vi "ClipCursor to PlotArea.vi"(7 "OriginPane":refnum<vi>, 8 "error in (no error)":errorcluster, 9 "VI":refnum<vi>, 10 "PlotPane":refnum<vi>, 11 "plot ref":refnum<vi>) -> (0 "error out":errorcluster)   [LabVIEW 2021, in "RocketPlot.lvlib"]
uses:
  RocketPlot.lvlib
  <vilib>/Utility/miscctls.llb/LVPointTypeDef.ctl
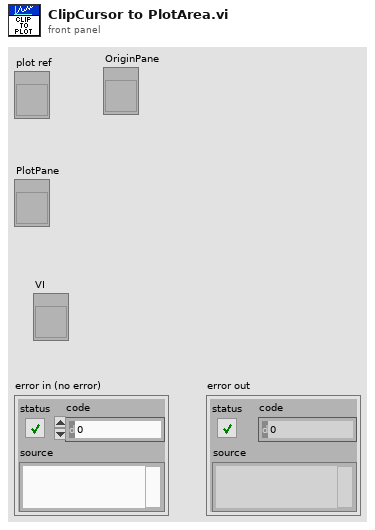
[diagram p1: front panel]
types:
  T1 = typedef "LVPointTypeDef.ctl" = cluster{"Horizontal":i16, "Vertical":i16}
  T2 = cluster{"Left":i32, "Top":i32, "Right":i32, "Bottom":i32}
  T3 = typedef "LVRectTypeDef.ctl" = cluster{"Left":i16, "Top":i16, "Right":i16, "Bottom":i16}
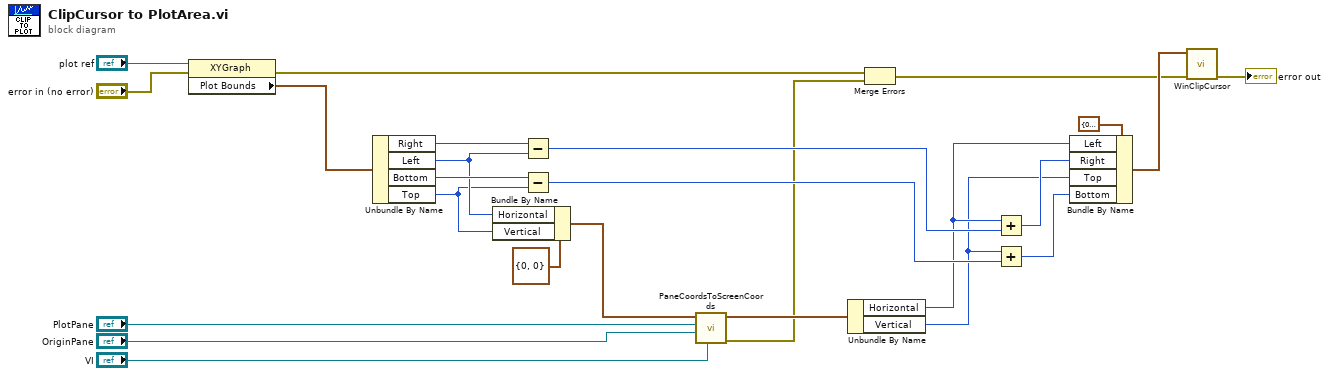
[diagram p0: block diagram]
diagram:
  n1 = property class="XYGraph"(reference="plot ref", error in="error in (no error)") -> (error out=w8:errorcluster, "Plot Bounds"=w24:T3)  [unwired: 1 out]
  n2 = Unbundle By Name(w24) -> ("Right"=w22:i16, "Left"=w16:i16, "Bottom"=w21:i16, "Top"=w15:i16)
  n3 = Bundle By Name(cluster=T1 {"Horizontal"=0, "Vertical"=0} ("Origin"), "Horizontal"=w16, "Vertical"=w15) -> (w6:T1)
  n4 = Subtract(x=w22, y=w16) -> (x-y=w20:i16)
  n5 = Subtract(x=w21, y=w15) -> (x-y=w18:i16)
  n6 = call "PaneCoordsToScreenCoords.vi"("VI"="VI", "Origin Pane"="OriginPane", "Owning Pane"="PlotPane", "Pane Coordinates"=w6) -> ("error out"=w1:errorcluster, "Screen Coords"=w2:T1)  [unwired: 6 in]
  n7 = Unbundle By Name(w2) -> ("Horizontal"=w10:i16, "Vertical"=w9:i16)
  n8 = Merge Errors(w8, w1) -> (w7:errorcluster)
  n9 = Add(x=w10, y=w20) -> (x+y=w19:i16)
  n10 = Add(x=w9, y=w18) -> (x+y=w17:i16)
  n11 = Bundle By Name(cluster=T2 {"Left"=0, "Top"=0, "Right"=0, "Bottom"=0} ("output cluster"), "Left"=w10, "Right"=w19, "Top"=w9, "Bottom"=w17) -> (w12:T2)
  n12 = call "WinClipCursor.vi"("error in (no error)"=w7, "RECT"=w12) -> ("error out"=→"error out":errorcluster)  [unwired: 9 in]
